vi "Mudule Input Check.vi"(9 "Data In":dbl, 11 "Value":T1) -> (3 "OK?":bool)   [LabVIEW 2020]
uses:
  Global/Data Global/SDQ Data Type.ctl
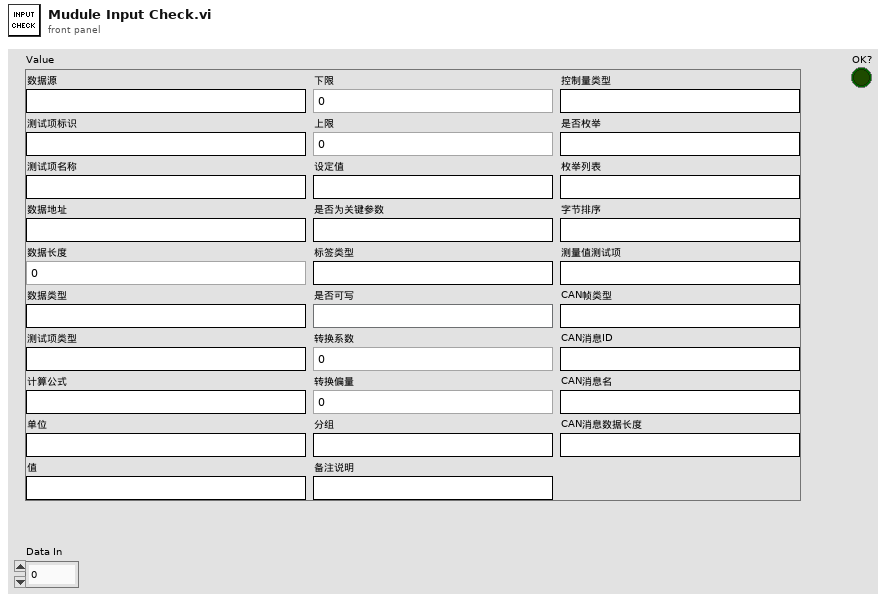
[diagram p1: front panel]
types:
  T1 = typedef "SDQ Data Type.ctl" = cluster{"CAN Length":string, "CAN Name":string, "CAN ID":string, "CAN Type":string, "Test Item":string, "Byte Order":string, "Instruction":string, "Control Type":string, "Group":string, "Offset":dbl, "Coefficient":dbl, "Write Enable":bool, "Lable Type":string, "Key?":string, "Set Value":string, "Upper":dbl, "Lower":dbl, "Unit":string, "Formula":string, "Test Item Type":string, "Length":i32, "Address":string, "Name":string, "Identifier":string, "Data Type":string, "Enumerate?":string, "Enumerate List":string, "Data":string, "Source":string}
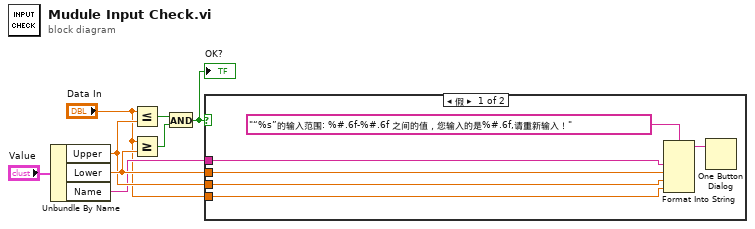
[diagram p0: block diagram]
diagram:
  n1 = Unbundle By Name("Value") -> ("Upper"=w4:dbl, "Lower"=w6:dbl, "Name"=w3:string)
  n2 = Less Or Equal?(x="Data In", y=w4) -> (x <= y?=w7:bool)
  n3 = Greater Or Equal?(x="Data In", y=w6) -> (x >= y?=w8:bool)
  n4 = And(x=w7, y=w8) -> (x .and. y?=w5:bool)
  "OK?" <- w5
  n5 = case shown="假" w5 {
    tunnel: w6 -> [w14 _]
    tunnel: w4 -> [w13 _]
    tunnel: w3 -> [w11 _]
    tunnel: "Data In" -> [w10 _]
    frame False {
      n6 = Format Into String(format string="“%s”的输入范围: %#.6f-%#.6f 之间的值，您输入的是%#.6f,请重新输入！" ("消息"), w11, w14, w13, w10) -> (resulting string=w12:string)  [unwired: 2 in, 1 out]
      n7 = One Button Dialog(message=w12) -> ()  [unwired: 1 in, 1 out]
    }
    frame True {
    }
  }
